vi "simulator_0720.vi"() -> ()   [LabVIEW 2017]
doc: "This example demonstrates how to continuously acquire buffered voltage measurements using a DAQmx device.\n\nFor instructions on how to connect your signals to the DAQ device, refer to your device documentation."
uses:
  <vilib>/Utility/error.llb/DialogType.ctl
  <vilib>/DAQmx/read.llb/DAQmx Read (Analog 1D Wfm NChan NSamp).vi
  <vilib>/DAQmx/configure/task.llb/DAQmx Configure Logging (TDMS).vi
  <vilib>/DAQmx/miscellaneous.llb/DAQmx Fill In Error Info.vi
  <vilib>/express/express shared/transition.llb/Dynamic To Waveform Array.vi
  <vilib>/express/express arith-compare/Formula/Block/exnFormulaBlock how many pts in the wave.vi
  <vilib>/express/express shared/ex_Modify Signal Name.vi
  <vilib>/express/express shared/transition.llb/Waveform Array To Dynamic.vi
  <vilib>/measure/maspectr.llb/FFT Power Spectrum and PSD for N Chan.vi
  <vilib>/express/express arith-compare/Formula/XNode/ExpressFormulaBlockNode.xnode
  <vilib>/measure/NI_MAPro.lvlib
  SetupDAQ.vi
panel:
  in  "Sensor C Channel 2":tag="Dev2/ai0"
  in  "Sensor D Channel 2":tag="Dev2/ai1"
  in  "Terminal config 2":i32(ring)=10083 items=["default"=-1, "RSE"=10083, "NRSE"=10078, "Differential"=10106, "Pseudodifferential"=12529]
  out "A,B Filtering Signal 2":dynamicdata(graph)
  out "55-65(A)":dynamicdata(graph)
  out "55-65(B)":dynamicdata(graph)
  out "10-20(B)":dynamicdata(graph)
  out "10-20(A)":dynamicdata(graph)
  out "A,B Original Signal 2":waveform(dbl)[](graph)
  out "웨이브폼 그래프":dynamicdata(graph)
  out "FFT Power Spectrum 2":dynamicdata(graph)
  out "A,B Filtering Signal":dynamicdata(graph)
  out "Sensor A Raw 5":dynamicdata(graph)
  in  "number of averages":u32=1
  out "Power Spectrum / PSD":cluster{"f0":dbl, "df":dbl, "magnitude":dbl[]}[](graph)
  out "detected amplitudes 2":dbl(graph)=1.1331379876254155
  out "detected frequencies 2":dbl(graph)=60.0
  out "detected frequencies":dbl[](array[numeric])=[60.0, 60.0]
  out "detected amplitudes":dbl[](array[numeric])=[1.1331379876254155, 0.40633237156802526]
  out "Sensor Raw 2":waveform(dbl)[](graph)
  out "Raw Signal":waveform(dbl)[](graph)
  in  "TDMS File Path":path
  in  "Logging Mode":i32(ring)=10231 items=["Off"=10231, "Log and Read"=15842]
  in  "Sensor B Channel":tag="Dev2/ai1"
  in  "Sensor A Channel":tag="Dev2/ai0"
  in  "Terminal config":i32(ring)=10083 items=["default"=-1, "RSE"=10083, "NRSE"=10078, "Differential"=10106, "Pseudodifferential"=12529]
  in  "rate":dbl=5000.0
  out "FFT Power Spectrum":cluster{"f0":dbl, "df":dbl, "magnitude":dbl[]}[](graph)
  in  "Stop":bool
  in  "Number of Samples":i32=100
  # "Channel Settings"
  # "Logging Settings"
  # "A-B Signal Display"
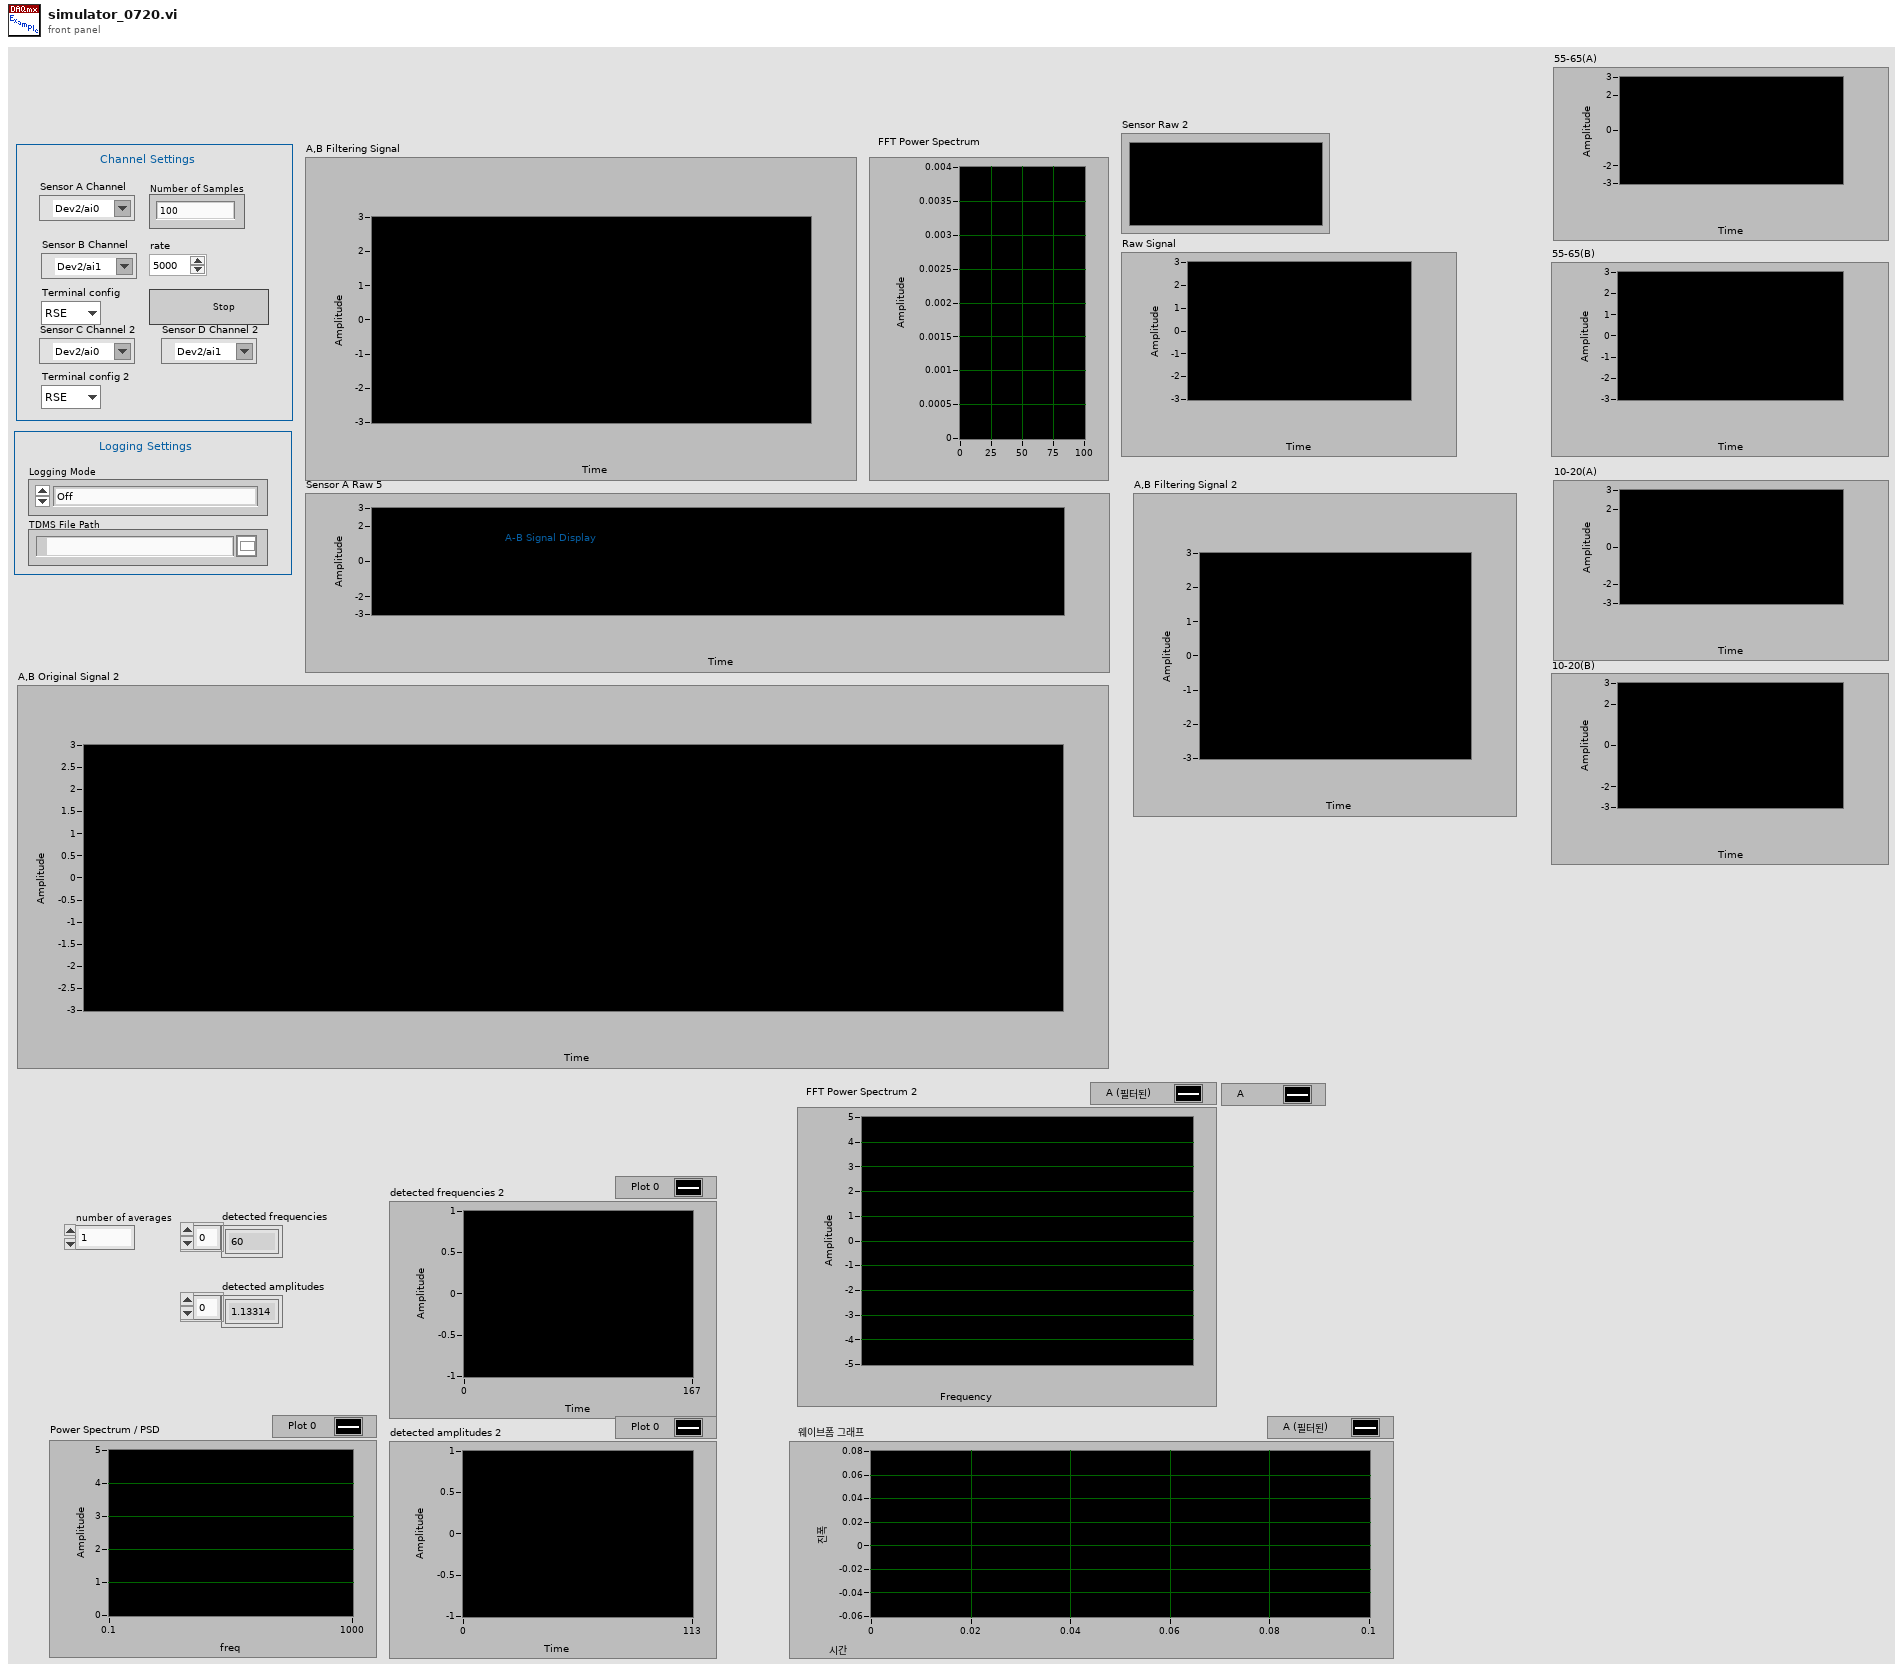
[diagram p1: front panel]
types:
  T1 = typedef "DialogType.ctl" = u16
  T2 = cluster{"averaging mode":enum16{"No averaging", "Vector averaging", "RMS averaging", "Peak hold"}, "weighting mode":enum16{"Linear", "Exponential"}, "number of averages":u32}
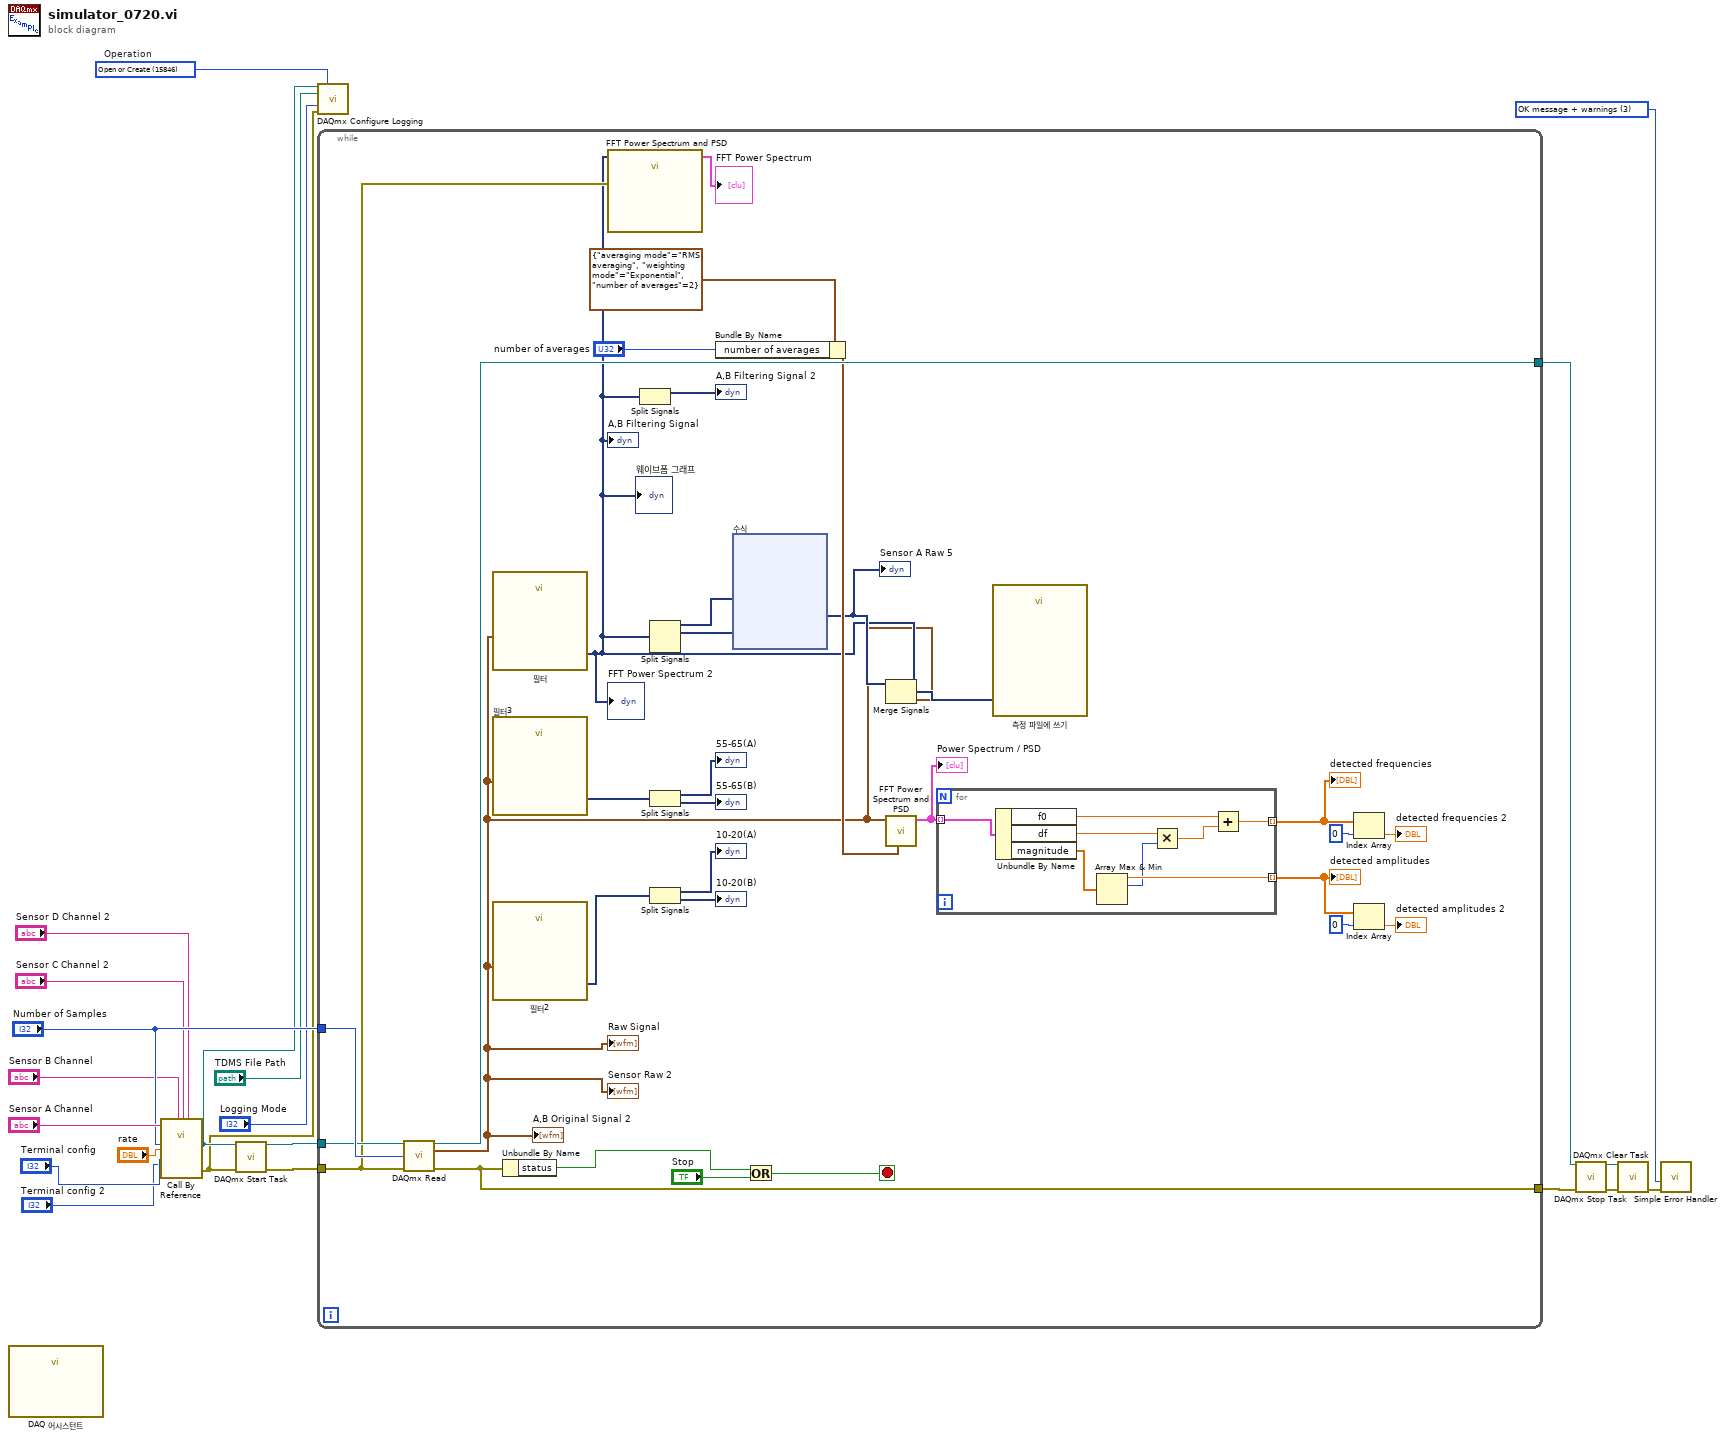
[diagram p0: block diagram]
diagram:
  w10 = 15846 items=["Open"=10437, "Open or Create"=15846, "Create or Replace"=15847, "Create"=15848]  # Operation
  w14 = T1 3 items=["no dialog", "OK message", "continue or stop message", "OK message + warnings", "continue/stop + warnings"] ("type of dialog (OK msg:1)")
  n1 = call "DAQ 어시스턴트"() -> ()  [unwired: 12 in]
  n2 = call-by-ref "?"("number of samples"="Number of Samples", "rate"="rate", "input terminal configuration"="Terminal config", "input terminal configuration 2"="Terminal config 2", "physical channel"="Sensor A Channel", "physical channel 2"="Sensor B Channel", "physical channel 3"="Sensor C Channel 2", "physical channel 4"="Sensor D Channel 2") -> ("task out"=w7:refnum<k21>, "error out"=w6:errorcluster)  [unwired: 12 in, 2 out]
  n3 = call <vilib>:"DAQmx Start Task.vi"("task/channels in"=w7, "error in"=w6) -> ("task out"=w21:refnum<k21>, "error out"=w20:errorcluster)  [unwired: 12 in]
  n4 = call-poly <vilib>:"DAQmx Configure Logging.vi"("task/channels in"=w7, "operation"=w10, "file path"="TDMS File Path", "logging mode"="Logging Mode", "error in"=w6) -> ()  [unwired: 9 in, 2 out]
  n5 = while {
    tunnel: w21 -> [w47]
    tunnel: w20 -> [w46]
    tunnel: [w53] -> w18
    tunnel: [w51] -> w17
    tunnel: "Number of Samples" -> [w48]
    stop <- w49 stop-if-true
    n6 = call-poly <vilib>:"DAQmx Read.vi"("task/channels in"=w47, "number of samples per channel"=w48, "error in"=w46) -> ("task out"=w53:refnum<k21>, "data"=w22:waveform(dbl)[], "error out"=w51:errorcluster)  [unwired: 10 in]
    "Raw Signal" <- w22
    "Sensor Raw 2" <- w22
    "A,B Original Signal 2" <- w22
    n7 = call "필터"("Signal"=w22) -> ("Filtered Signal"=w23:dynamicdata)  [unwired: 9 in, 1 out]
    "A,B Filtering Signal" <- w23
    "FFT Power Spectrum 2" <- w23
    "웨이브폼 그래프" <- w23
    n8 = call "필터3"("Signal"=w22) -> ("Filtered Signal"=w28:dynamicdata)  [unwired: 9 in, 1 out]
    n9 = call "필터2"("Signal"=w22) -> ("Filtered Signal"=w33:dynamicdata)  [unwired: 9 in, 1 out]
    n10 = Unbundle By Name(w51) -> ("status"=w50:bool)
    n11 = call-poly <vilib>:"FFT Power Spectrum and PSD.vi"("error in (no error)"=w46, "time signals"=w23) -> ("Power Spectrum / PSD"=→"FFT Power Spectrum":cluster{"f0":dbl, "df":dbl, "magnitude":dbl[]}[])  [unwired: 6 in, 3 out]
    n12 = Split Signals(w23) -> (→"A,B Filtering Signal 2":dynamicdata)  [unwired: 2 in, 1 out]
    n13 = Split Signals(w23) -> (w25:dynamicdata, w24:dynamicdata)  [unwired: 4 in, 2 out]
    n14 = Split Signals(w28) -> (→"55-65(A)":dynamicdata, →"55-65(B)":dynamicdata)  [unwired: 2 in]
    n15 = Split Signals(w33) -> (→"10-20(A)":dynamicdata, →"10-20(B)":dynamicdata)  [unwired: 2 in]
    n16 = Bundle By Name(cluster=T2 {"averaging mode"=enum."RMS averaging", "weighting mode"=enum."Exponential", "number of averages"=2} ("averaging parameters"), "number of averages"="number of averages") -> (w37:T2)
    n17 = xnode "수식"("X1"=w25, "X2"=w24) -> ("결과"=w26:dynamicdata)  [unwired: 1 in, 1 out]
    "Sensor A Raw 5" <- w26
    n18 = Or(x=w50, y="Stop") -> (x .or. y?=w49:bool)
    n19 = Merge Signals(w26, w23, w22) -> (w34:dynamicdata)
    n20 = call-poly <vilib>:"FFT Power Spectrum and PSD.vi"("averaging parameters"=w37, "time signals"=w22) -> ("Power Spectrum / PSD"=w44:cluster{"f0":dbl, "df":dbl, "magnitude":dbl[]}[])  [unwired: 6 in, 3 out]
    "Power Spectrum / PSD" <- w44
    n21 = for {
      tunnel: w44 -> [w61] mode=indexing
      tunnel: [w59] -> w42 mode=indexing
      tunnel: [w54] -> w39 mode=indexing
      n22 = Unbundle By Name(w61) -> ("f0"=w58:dbl, "df"=w55:dbl, "magnitude"=w60:dbl[])
      n23 = Array Max & Min(array=w60) -> (max value=w59:dbl, max index (indices)=w56:i32)  [unwired: 2 out]
      n24 = Multiply(x=w55, y=w56) -> (x*y=w57:dbl)
      n25 = Add(x=w58, y=w57) -> (x+y=w54:dbl)
    }
    "detected amplitudes" <- w42
    "detected frequencies" <- w39
    n26 = call "측정 파일에 쓰기"("Signals"=w34) -> ()  [unwired: 16 in, 3 out]
    n27 = Index Array(array=w39, index=0) -> (element=→"detected frequencies 2":dbl)
    n28 = Index Array(array=w42, index=0) -> (element=→"detected amplitudes 2":dbl)
  }
  n29 = call <vilib>:"DAQmx Stop Task.vi"("task/channels in"=w18, "error in"=w17) -> ("task out"=w15:refnum<k21>, "error out"=w16:errorcluster)  [unwired: 12 in]
  n30 = call <vilib>:"DAQmx Clear Task.vi"("task in"=w15, "error in"=w16) -> ("error out"=w19:errorcluster)  [unwired: 13 in]
  n31 = call <vilib>:"Simple Error Handler.vi"("type of dialog (OK msg:1)"=w14, "error in (no error)"=w19) -> ()  [unwired: 3 in, 5 out]
